vi "Server send.vi"() -> ()   [LabVIEW 2016, in "自动更新.lvlib" / "TCP文件传输系统.lvlib"]
uses:
  <vilib>/Utility/miscctls.llb/LVPointTypeDef.ctl
  <vilib>/Utility/sysdir.llb/System Directory Type.ctl
  <vilib>/Averna/Notify Icon/NotifyIcon.llb/BalloonIcon.ctl
  <vilib>/Averna/Notify Icon/NotifyIcon.llb/GetSelectedItemEvent.vi
  <vilib>/Averna/Notify Icon/NotifyIcon.llb/SetVisible.vi
  <vilib>/Averna/Notify Icon/NotifyIcon.llb/SetMenuDefaultItem.vi
  <vilib>/Averna/Notify Icon/NotifyIcon.llb/SetTipText.vi
  <vilib>/Averna/Notify Icon/NotifyIcon.llb/NotifyIcon.lvclass
panel:
  in  "选项卡控件 2":enum32{"数据传输系统", "固定站系统"}(tab)
  in  "选项卡控件":T1(tab)
  out "TCP发送全局簇":T2
  out "文件传输的路径":path
  in  "Application":string="版本升级文档.txt"
  in  "远程端口或服务名称":u16=11235
  out "本机网络地址":string="192.168.1.250"
  out "TCP发送全局簇 2":T2
  out "文件传输的路径 2":path
  in  "Application 2":string="update.exe"
  in  "远程端口或服务名称 2":u16=11236
  out "本机网络地址 2":string="192.168.1.250"
  out "TCP发送全局簇 3":T2
  out "文件传输的路径 3":path
  in  "Application 3":string="平台数据传输系统.exe"
  in  "远程端口或服务名称 3":u16=11234
  out "本机网络地址 3":string="192.168.1.250"
  in  "选项卡控件 3":enum32{"固定站版本txt", "固定站update", "固定站exe"}(tab)
  in  "Application 5":string="版本升级文档.txt"
  out "TCP发送全局簇 5":T2
  out "本机网络地址 5":string="192.168.1.250"
  in  "远程端口或服务名称 5":u16=10051
  out "文件传输的路径 5":path
  out "文件传输的路径 6":path
  in  "远程端口或服务名称 6":u16=10052
  out "本机网络地址 6":string="192.168.1.250"
  out "TCP发送全局簇 6":T2
  in  "Application 6":string="update.exe"
  in  "Application 4":string="一体化水质自动监测系统.exe"
  out "TCP发送全局簇 4":T2
  out "本机网络地址 4":string="192.168.1.250"
  in  "远程端口或服务名称 4":u16=10050
  out "文件传输的路径 4":path
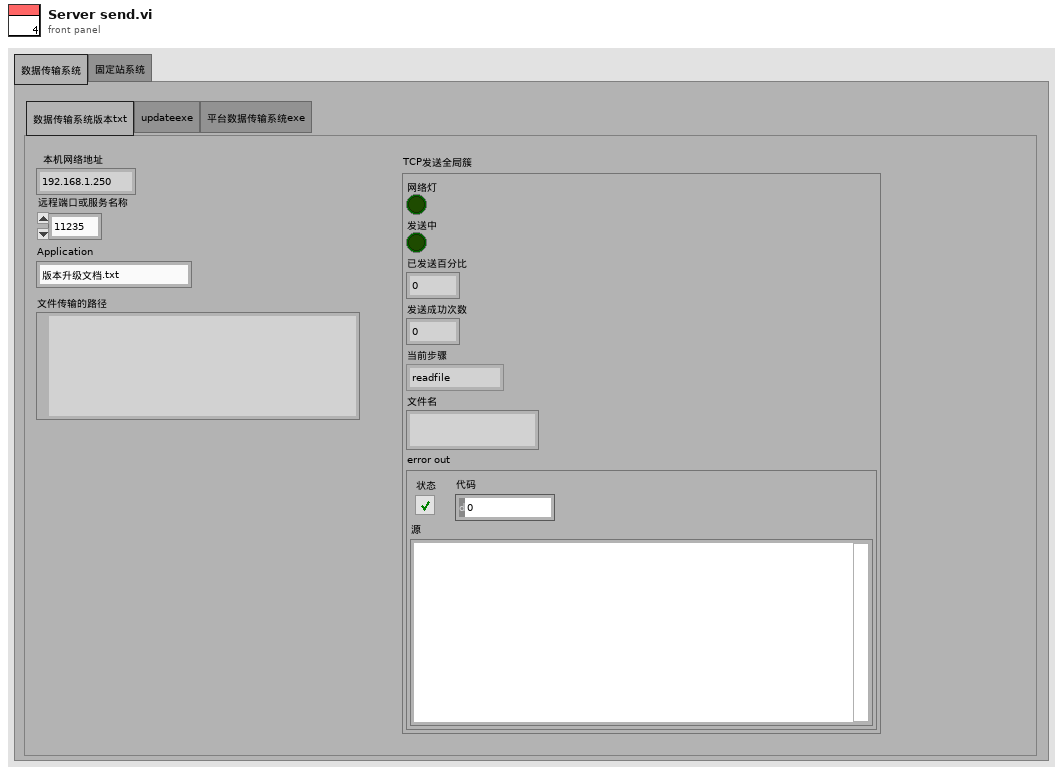
[diagram p1: front panel]
types:
  T1 = enum32{"数据传输系统版本txt", "updateexe", "平台数据传输系统exe"}
  T2 = cluster{"网络灯":bool, "发送中":bool, "已发送百分比":u8, "发送成功次数":dbl, "当前步骤":enum16{"readfile", "init", "sendhead", "sendcontent", "sendsuccess", "over"}, "文件名":string, "error out":errorcluster}
  T3 = enum32{"Invalid", "Standard", "Closed", "Hidden", "Minimized", "Maximized"}
  T4 = typedef "LVPointTypeDef.ctl" = cluster{"Horizontal":i16, "Vertical":i16}
  T5 = typedef "NotifyIcon.lvlib/NotifyIcon.lvclass/BalloonIcon.ctl" = enum32{"None", "Information", "Warning", "Error"}
  T6 = typedef "System Directory Type.ctl" = i32
  T7 = enum32{"invalid app kind", "Development System", "Run Time System", "Student Edition", "Embedded LabVIEW", "Evaluation", "Custom"}
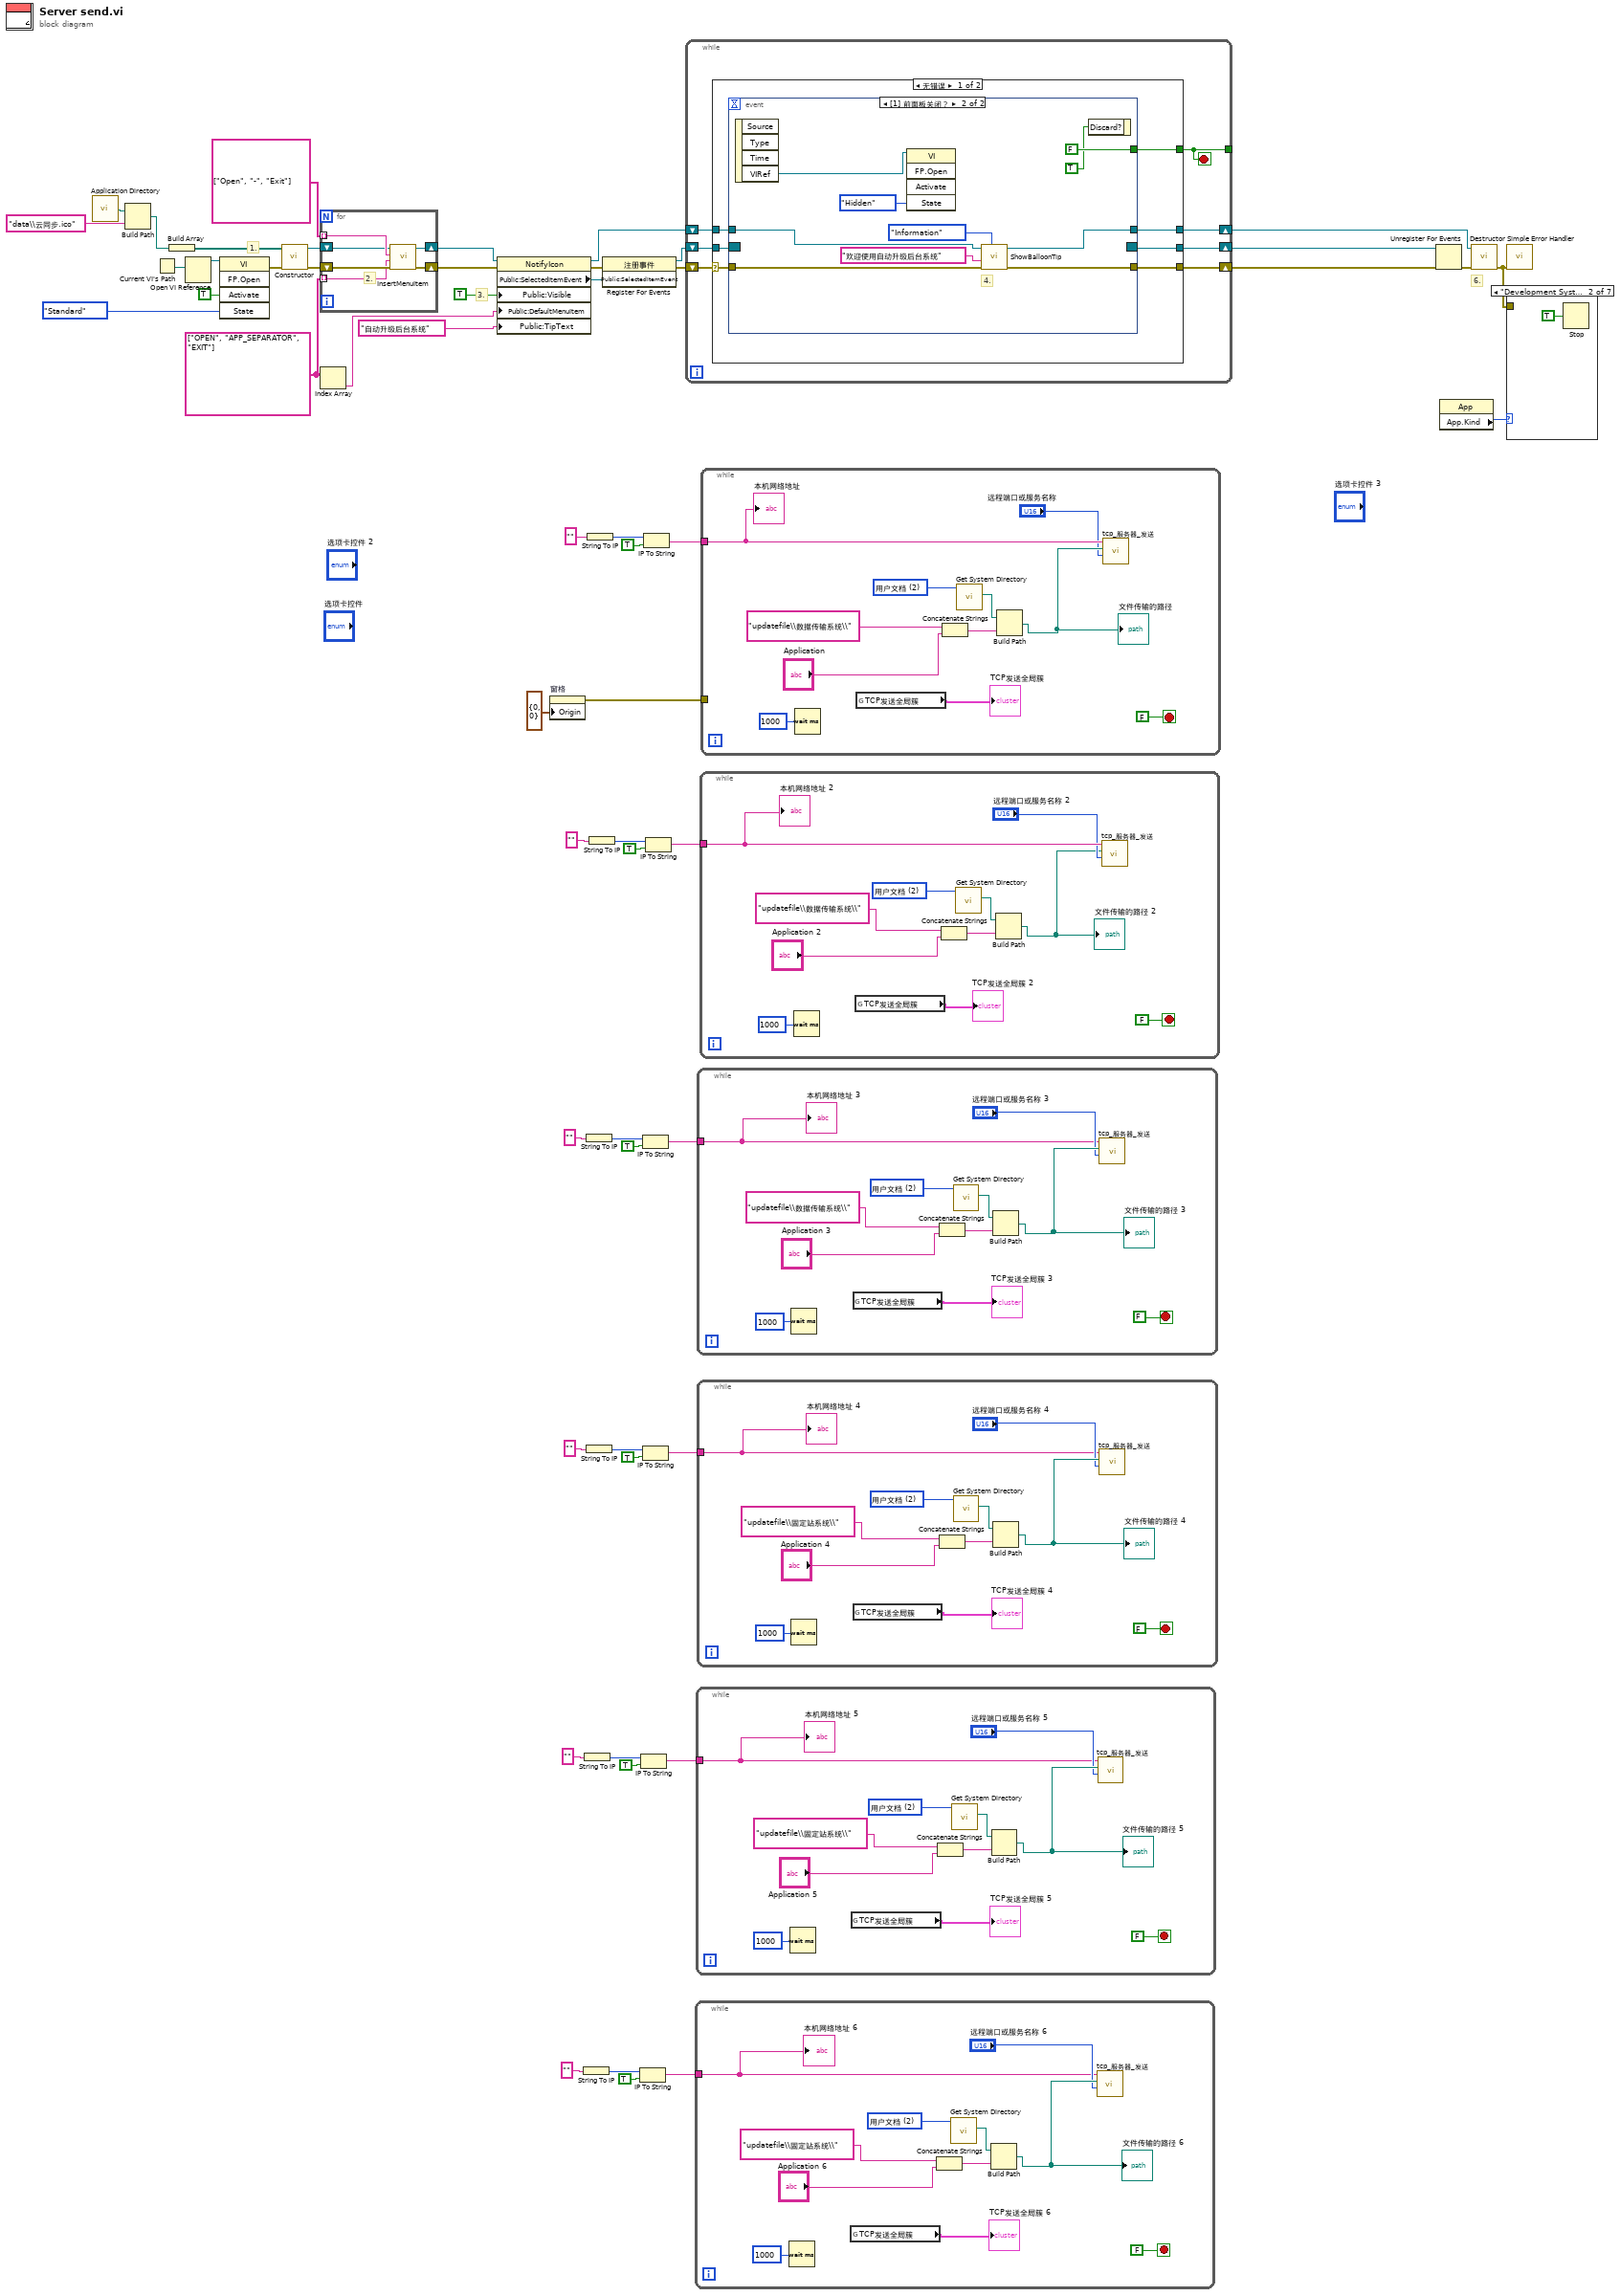
[diagram p0: block diagram]
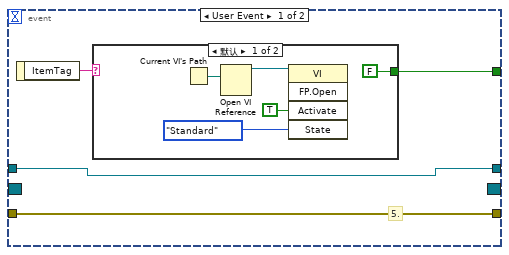
[diagram p2: hidden frame]
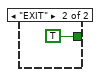
[diagram p3: hidden frame]
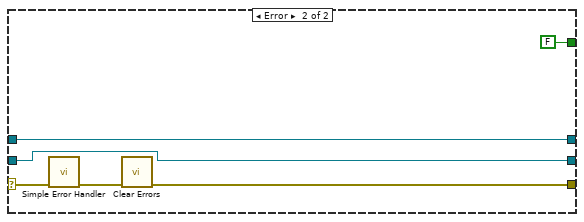
[diagram p4: hidden frame]
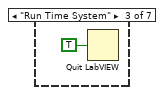
[diagram p6: hidden frame]
diagram:
  w25 = string[] ["OPEN", "APP_SEPARATOR", "EXIT"]
  # "6."
  # "3."
  # "1."
  n1 = call <vilib>:"Application Directory.vi"() -> ("Application Directory"=w23:path)
  n2 = Build Path(base path=w23, name or relative path="data\\云同步.ico" ("名称或相对路径")) -> (appended path=w33:path)
  n3 = Current VI's Path() -> (path=w20:path)
  n4 = Build Array(w33) -> (w28:path[])
  n5 = Open VI Reference(vi path=w20) -> (vi reference=w19:refnum<vi>)  [unwired: 5 in, 1 out]
  n6 = invoke class="VI" method="FP.Open"(reference=w19, "Activate"=TRUE ("激活？"), "State"=T3."Standard" ("状态")) -> (error out=w18:errorcluster)  [unwired: 2 in, 4 out]
  n7 = call <vilib>:"Constructor.vi"("error in"=w18, "IconFilePathList"=w28) -> ("error out"=w32:errorcluster, "NotifyIcon"=w24:refnum<class "NotifyIcon.lvclass">)  [unwired: 8 in]
  n8 = for {
    shift-right: [w60] -> w43
    shift-left: w32 -> [w61]
    tunnel: string[] ["Open", "-", "Exit"] -> [w59] mode=indexing
    tunnel: w25 -> [w58] mode=indexing
    shift-right: [w56] -> w42
    shift-left: w24 -> [w57]
    # "2."
    n9 = call <vilib>:"InsertMenuItem.vi"("error in"=w61, "ItemTag"=w58, "ItemName"=w59, "NotifyIcon in"=w57) -> ("error out"=w60:errorcluster, "NotifyIcon out"=w56:refnum<class "NotifyIcon.lvclass">)  [unwired: 6 in]
  }
  n10 = Index Array(array=w25) -> (element=w26:string)  [unwired: 1 in]
  n11 = property class="NotifyIcon"(reference=w42, error in=w43, "Public:Visible"=TRUE ("Visible"), "Public:DefaultMenuItem"=w26, "Public:TipText"="自动升级后台系统" ("TipText")) -> (reference out=w39:refnum<class "NotifyIcon.lvclass">, error out=w31:errorcluster, "Public:SelectedItemEvent"=w30:refnum<user-event>)
  n12 = property on="窗格" class="Pane"("Origin"=T4 {"Horizontal"=0, "Vertical"=0} ("原点")) -> (error out=w13:errorcluster)  [unwired: 2 in, 1 out]
  n13 = String To IP(1:"" ("名称")) -> (0:w2:u32)
  n14 = String To IP(1:"" ("名称")) -> (0:w7:u32)
  n15 = String To IP(1:"" ("名称")) -> (0:w46:u32)
  n16 = String To IP(1:"" ("名称")) -> (0:w10:u32)
  n17 = String To IP(1:"" ("名称")) -> (0:w53:u32)
  n18 = String To IP(1:"" ("名称")) -> (0:w49:u32)
  n19 = register-events(error in=w31, w30) -> (reference out=w15:refnum<event-registration>, error out=w16:errorcluster)  [unwired: 1 in]
  n20 = IP To String(1:TRUE ("句点符号？(F)"), 2:w2) -> (0:w1:string)
  n21 = IP To String(1:TRUE ("句点符号？(F)"), 2:w7) -> (0:w8:string)
  n22 = IP To String(1:TRUE ("句点符号？(F)"), 2:w46) -> (0:w47:string)
  n23 = IP To String(1:TRUE ("句点符号？(F)"), 2:w10) -> (0:w9:string)
  n24 = IP To String(1:TRUE ("句点符号？(F)"), 2:w53) -> (0:w52:string)
  n25 = IP To String(1:TRUE ("句点符号？(F)"), 2:w49) -> (0:w48:string)
  n26 = while {
    shift-right: [w65] -> w37
    shift-left: w16 -> [w64]
    shift-right: [w66] -> w35
    shift-left: w39 -> [w67]
    shift-right: [w63] -> w36
    shift-left: w15 -> [w68]
    tunnel: [w62] -> _
    stop <- w62 stop-if-true
    n27 = case shown="无错误" w64 {
      selector: w64 -> [w70 w101]
      tunnel: w68 -> [w75 w96]
      tunnel: w67 -> [w74 w97]
      tunnel: [w73 w97] -> w66
      tunnel: [w72 w99] -> w65
      tunnel: [w71 FALSE ("Discard?")] -> w62
      tunnel: [w69 w96] -> w63
      frame No Error {
        n28 = event shown="[1] 前面板关闭？" {
          selector: w75 -> [_ _]
          dyn-events: [_ _] -> w69
          timeout: _ -> [_ _]
          tunnel: w70 -> [w78 w94]
          tunnel: [w78 w93] -> w72
          tunnel: [w77 FALSE ("Discard?")] -> w71
          tunnel: w74 -> [w76 w95]
          tunnel: [w76 w92] -> w73
          event User Event {
            # "5."
            n29 = event-data() -> ("ItemTag"=w79:string)  [unwired: 1 in]
            n30 = case shown="默认" w79 {
              tunnel: [FALSE TRUE] -> w77
              frame Default {
                n31 = Current VI's Path() -> (path=w81:path)
                n32 = Open VI Reference(vi path=w81) -> (vi reference=w82:refnum<vi>)  [unwired: 5 in, 1 out]
                n33 = invoke class="VI" method="FP.Open"(reference=w82, "Activate"=TRUE ("激活？"), "State"=T3."Standard" ("状态")) -> ()  [unwired: 2 in, 5 out]
              }
              frame "EXIT" {
              }
            }
          }
          event Panel Close? {
            # "4."
            n34 = event-data() -> ("VIRef"=w88:refnum<vi>)  [unwired: 1 in, 3 out]
            n35 = invoke class="VI" method="FP.Open"(reference=w88, "State"=T3."Hidden" ("状态")) -> ()  [unwired: 3 in, 5 out]
            n36 = call <vilib>:"ShowBalloonTip.vi"("Balloon Icon"=BalloonIcon."Information", "error in"=w94, "Text"="欢迎使用自动升级后台系统", "NotifyIcon in"=w95) -> ("error out"=w93:errorcluster, "NotifyIcon out"=w92:refnum<class "NotifyIcon.lvclass">)  [unwired: 6 in]
            n37 = event-data("Discard?"=TRUE ("放弃？")) -> ()  [unwired: 1 in, 1 out]
          }
        }
      }
      frame Error {
        n38 = call <vilib>:"Simple Error Handler.vi"("error in (no error)"=w101) -> ("error out"=w100:errorcluster)  [unwired: 4 in, 4 out]
        n39 = call <vilib>:"Clear Errors.vi"("error in (no error)"=w100) -> ("error out"=w99:errorcluster)  [unwired: 5 in, 1 out]
      }
    }
  }
  n40 = while {
    tunnel: w1 -> [w105]
    stop <- FALSE stop-if-true
    w111 = T6 2 items=["用户目录"=0, "用户桌面"=1, "用户文档"=2, "用户应用程序数据"=3, "用户设置"=4, "用户临时目录"=5, "公共文档"=6, "公共应用程序数据"=7, "公共设置"=8, "公共缓存"=13, "系统核心库"=9, "系统安装库"=10, "应用程序文件"=11, "启动盘根目录"=12] ("system directory type")
    n41 = Wait (ms)(milliseconds to wait=u32 1000 ("等待时间（毫秒）")) -> ()  [unwired: 1 out]
    n42 = global read "全局变量1.vi" "TCP发送全局簇"() -> (→"TCP发送全局簇 6":T2)
    n43 = Concatenate Strings("updatefile\\固定站系统\\" ("condition"), "Application 6") -> (w110:string)
    n44 = call <vilib>:"Get System Directory.vi"("system directory type"=w111) -> ("system directory"=w109:path)  [unwired: 10 in]
    n45 = Build Path(base path=w109, name or relative path=w110) -> (appended path=w107:path)
    "文件传输的路径 6" <- w107
    n46 = call "tcp_服务器_发送.vi"("远程端口或服务名称"="远程端口或服务名称 6", "原文件路径（使用对话框）"=w107, "服务器网络地址"=w105) -> ()  [unwired: 9 in]
    "本机网络地址 6" <- w105
  }
  n47 = while {
    tunnel: w8 -> [w116]
    stop <- FALSE stop-if-true
    w122 = T6 2 items=["用户目录"=0, "用户桌面"=1, "用户文档"=2, "用户应用程序数据"=3, "用户设置"=4, "用户临时目录"=5, "公共文档"=6, "公共应用程序数据"=7, "公共设置"=8, "公共缓存"=13, "系统核心库"=9, "系统安装库"=10, "应用程序文件"=11, "启动盘根目录"=12] ("system directory type")
    n48 = Wait (ms)(milliseconds to wait=u32 1000 ("等待时间（毫秒）")) -> ()  [unwired: 1 out]
    n49 = global read "全局变量1.vi" "TCP发送全局簇"() -> (→"TCP发送全局簇 5":T2)
    n50 = Concatenate Strings("updatefile\\固定站系统\\" ("condition"), "Application 5") -> (w121:string)
    n51 = call <vilib>:"Get System Directory.vi"("system directory type"=w122) -> ("system directory"=w120:path)  [unwired: 10 in]
    n52 = Build Path(base path=w120, name or relative path=w121) -> (appended path=w118:path)
    "文件传输的路径 5" <- w118
    n53 = call "tcp_服务器_发送.vi"("远程端口或服务名称"="远程端口或服务名称 5", "原文件路径（使用对话框）"=w118, "服务器网络地址"=w116) -> ()  [unwired: 9 in]
    "本机网络地址 5" <- w116
  }
  n54 = while {
    tunnel: w47 -> [w127]
    stop <- FALSE stop-if-true
    w133 = T6 2 items=["用户目录"=0, "用户桌面"=1, "用户文档"=2, "用户应用程序数据"=3, "用户设置"=4, "用户临时目录"=5, "公共文档"=6, "公共应用程序数据"=7, "公共设置"=8, "公共缓存"=13, "系统核心库"=9, "系统安装库"=10, "应用程序文件"=11, "启动盘根目录"=12] ("system directory type")
    n55 = Wait (ms)(milliseconds to wait=u32 1000 ("等待时间（毫秒）")) -> ()  [unwired: 1 out]
    n56 = global read "全局变量1.vi" "TCP发送全局簇"() -> (→"TCP发送全局簇 3":T2)
    n57 = Concatenate Strings("updatefile\\数据传输系统\\" ("condition"), "Application 3") -> (w132:string)
    n58 = call <vilib>:"Get System Directory.vi"("system directory type"=w133) -> ("system directory"=w131:path)  [unwired: 10 in]
    n59 = Build Path(base path=w131, name or relative path=w132) -> (appended path=w129:path)
    "文件传输的路径 3" <- w129
    n60 = call "tcp_服务器_发送.vi"("远程端口或服务名称"="远程端口或服务名称 3", "原文件路径（使用对话框）"=w129, "服务器网络地址"=w127) -> ()  [unwired: 9 in]
    "本机网络地址 3" <- w127
  }
  n61 = while {
    tunnel: w9 -> [w138]
    stop <- FALSE stop-if-true
    w144 = T6 2 items=["用户目录"=0, "用户桌面"=1, "用户文档"=2, "用户应用程序数据"=3, "用户设置"=4, "用户临时目录"=5, "公共文档"=6, "公共应用程序数据"=7, "公共设置"=8, "公共缓存"=13, "系统核心库"=9, "系统安装库"=10, "应用程序文件"=11, "启动盘根目录"=12] ("system directory type")
    n62 = Wait (ms)(milliseconds to wait=u32 1000 ("等待时间（毫秒）")) -> ()  [unwired: 1 out]
    n63 = global read "全局变量1.vi" "TCP发送全局簇"() -> (→"TCP发送全局簇 4":T2)
    n64 = Concatenate Strings("updatefile\\固定站系统\\" ("condition"), "Application 4") -> (w143:string)
    n65 = call <vilib>:"Get System Directory.vi"("system directory type"=w144) -> ("system directory"=w142:path)  [unwired: 10 in]
    n66 = Build Path(base path=w142, name or relative path=w143) -> (appended path=w140:path)
    "文件传输的路径 4" <- w140
    n67 = call "tcp_服务器_发送.vi"("远程端口或服务名称"="远程端口或服务名称 4", "原文件路径（使用对话框）"=w140, "服务器网络地址"=w138) -> ()  [unwired: 9 in]
    "本机网络地址 4" <- w138
  }
  n68 = while {
    tunnel: w48 -> [w151]
    stop <- FALSE stop-if-true
    w155 = T6 2 items=["用户目录"=0, "用户桌面"=1, "用户文档"=2, "用户应用程序数据"=3, "用户设置"=4, "用户临时目录"=5, "公共文档"=6, "公共应用程序数据"=7, "公共设置"=8, "公共缓存"=13, "系统核心库"=9, "系统安装库"=10, "应用程序文件"=11, "启动盘根目录"=12] ("system directory type")
    n69 = Wait (ms)(milliseconds to wait=u32 1000 ("等待时间（毫秒）")) -> ()  [unwired: 1 out]
    n70 = global read "全局变量1.vi" "TCP发送全局簇"() -> (→"TCP发送全局簇 2":T2)
    n71 = Concatenate Strings("updatefile\\数据传输系统\\" ("condition"), "Application 2") -> (w154:string)
    n72 = call <vilib>:"Get System Directory.vi"("system directory type"=w155) -> ("system directory"=w153:path)  [unwired: 10 in]
    n73 = Build Path(base path=w153, name or relative path=w154) -> (appended path=w147:path)
    "文件传输的路径 2" <- w147
    n74 = call "tcp_服务器_发送.vi"("远程端口或服务名称"="远程端口或服务名称 2", "原文件路径（使用对话框）"=w147, "服务器网络地址"=w151) -> ()  [unwired: 9 in]
    "本机网络地址 2" <- w151
  }
  n75 = while {
    tunnel: w52 -> [w165]
    tunnel: w13 -> [_]
    stop <- FALSE stop-if-true
    w166 = T6 2 items=["用户目录"=0, "用户桌面"=1, "用户文档"=2, "用户应用程序数据"=3, "用户设置"=4, "用户临时目录"=5, "公共文档"=6, "公共应用程序数据"=7, "公共设置"=8, "公共缓存"=13, "系统核心库"=9, "系统安装库"=10, "应用程序文件"=11, "启动盘根目录"=12] ("system directory type")
    n76 = Wait (ms)(milliseconds to wait=u32 1000 ("等待时间（毫秒）")) -> ()  [unwired: 1 out]
    n77 = global read "全局变量1.vi" "TCP发送全局簇"() -> (→"TCP发送全局簇":T2)
    n78 = Concatenate Strings("updatefile\\数据传输系统\\" ("condition"), "Application") -> (w164:string)
    n79 = call <vilib>:"Get System Directory.vi"("system directory type"=w166) -> ("system directory"=w162:path)  [unwired: 10 in]
    n80 = Build Path(base path=w162, name or relative path=w164) -> (appended path=w161:path)
    "文件传输的路径" <- w161
    n81 = call "tcp_服务器_发送.vi"("远程端口或服务名称"="远程端口或服务名称", "原文件路径（使用对话框）"=w161, "服务器网络地址"=w165) -> ()  [unwired: 9 in]
    "本机网络地址" <- w165
  }
  n82 = Unregister For Events(event registration refnum=w36, error in=w37) -> (error out=w38:errorcluster)
  n83 = property class="App"() -> ("App.Kind"=w17:T7)  [unwired: 2 in, 2 out]
  n84 = call <vilib>:"Destructor.vi"("error in"=w38, "NotifyIcon"=w35) -> ("error out"=w34:errorcluster)  [unwired: 9 in]
  n85 = call <vilib>:"Simple Error Handler.vi"("error in (no error)"=w34) -> ()  [unwired: 4 in, 5 out]
  n86 = case shown="\"Development System\"" w17 {
    tunnel: w34 -> [_ _ _ _ _ _ _]
    frame "invalid app kind", Default {
    }
    frame "Development System" {
      n87 = Stop(stop? (T)=TRUE ("可见")) -> ()
    }
    frame "Run Time System" {
      n88 = Quit LabVIEW(quit? (T)=TRUE ("退出？(T)")) -> ()
    }
    frame "Student Edition" {
    }
    frame "Embedded LabVIEW" {
    }
    frame "Evaluation" {
    }
    frame "Custom" {
    }
  }
